vi "SubVI_Medicao.vi"(0 "Osciloscópio":refnum<visa-resource-name>="GPIB0::1::INSTR") -> (1 "Osciloscópio out":refnum<visa-resource-name>, 2 "Vmax":dbl, 3 "Vmin":dbl, 4 "Fase":dbl)   [LabVIEW 2021]
uses:
  384dc7f3-02c4-4d01-8472-58ff4c9df96a.vi
  292b6b08-2108-49e1-b5db-6c0617326701.vi
  c9bba13f-fd71-44bd-afed-ce225723edfd.vi
  4dd9f0b6-0c3f-4367-96f8-2e699b3ef568.vi
  dfb05754-934e-4608-8b12-f2cc72ba2c6f.vi
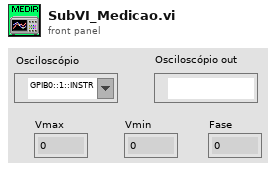
[diagram p1: front panel]
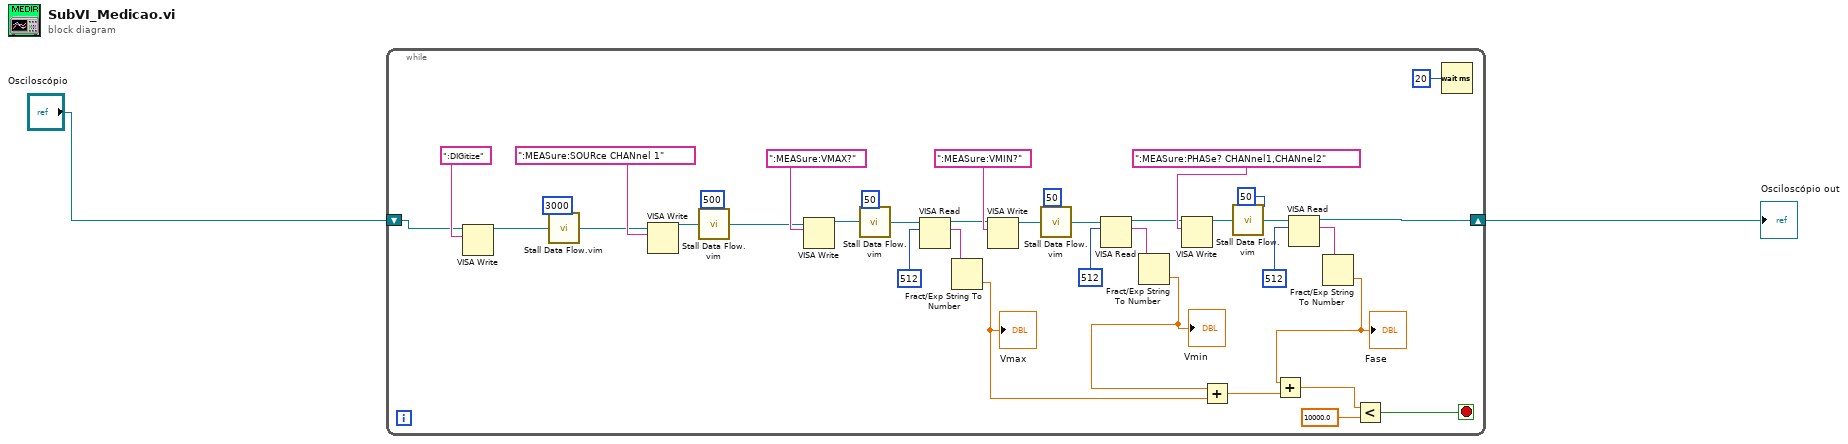
[diagram p0: block diagram]
diagram:
  n1 = while {
    shift-right: [w15] -> w2
    shift-left: "Osciloscópio" -> [w4]
    stop <- w24 stop-if-true
    n2 = VISA Write(VISA resource name=w4, write buffer=":DIGitize") -> (VISA resource name out=w5:refnum<visa-resource-name>)  [unwired: 1 in, 2 out]
    n3 = call "Stall Data Flow.vim"("value in"=w5, "milliseconds to wait"=u32 3000) -> ("value out"=w10:refnum<visa-resource-name>)  [unwired: 1 out]
    n4 = VISA Write(VISA resource name=w10, write buffer=":MEASure:SOURce CHANnel 1") -> (VISA resource name out=w7:refnum<visa-resource-name>)  [unwired: 1 in, 2 out]
    n5 = call "Stall Data Flow.vim"("value in"=w7, "milliseconds to wait"=u32 500) -> ("value out"=w3:refnum<visa-resource-name>)  [unwired: 1 out]
    n6 = VISA Write(VISA resource name=w3, write buffer=":MEASure:VMAX?") -> (VISA resource name out=w31:refnum<visa-resource-name>)  [unwired: 1 in, 2 out]
    n7 = call "Stall Data Flow.vim"("value in"=w31, "milliseconds to wait"=u32 50) -> ("value out"=w30:refnum<visa-resource-name>)  [unwired: 1 out]
    n8 = VISA Read(VISA resource name=w30, byte count=u32 512) -> (VISA resource name out=w36:refnum<visa-resource-name>, read buffer=w35:string)  [unwired: 1 in, 2 out]
    n9 = Fract/Exp String To Number(string=w35) -> (number=w26:dbl)  [unwired: 3 in, 1 out]
    "Vmax" <- w26
    n10 = VISA Write(VISA resource name=w36, write buffer=":MEASure:VMIN?") -> (VISA resource name out=w29:refnum<visa-resource-name>)  [unwired: 1 in, 2 out]
    n11 = call "Stall Data Flow.vim"("value in"=w29, "milliseconds to wait"=u32 50) -> ("value out"=w28:refnum<visa-resource-name>)  [unwired: 1 out]
    n12 = VISA Read(VISA resource name=w28, byte count=u32 512) -> (VISA resource name out=w16:refnum<visa-resource-name>, read buffer=w34:string)  [unwired: 1 in, 2 out]
    n13 = Fract/Exp String To Number(string=w34) -> (number=w27:dbl)  [unwired: 3 in, 1 out]
    "Vmin" <- w27
    n14 = VISA Write(VISA resource name=w16, write buffer=":MEASure:PHASe? CHANnel1,CHANnel2") -> (VISA resource name out=w22:refnum<visa-resource-name>)  [unwired: 1 in, 2 out]
    n15 = Add(x=w27, y=w26) -> (x+y=w14:dbl)
    n16 = call "Stall Data Flow.vim"("value in"=w22, "milliseconds to wait"=u32 50) -> ("value out"=w21:refnum<visa-resource-name>)  [unwired: 1 out]
    n17 = VISA Read(VISA resource name=w21, byte count=u32 512) -> (VISA resource name out=w15:refnum<visa-resource-name>, read buffer=w20:string)  [unwired: 1 in, 2 out]
    n18 = Fract/Exp String To Number(string=w20) -> (number=w13:dbl)  [unwired: 3 in, 1 out]
    "Fase" <- w13
    n19 = Add(x=w13, y=w14) -> (x+y=w12:dbl)
    n20 = Less?(x=w12, y=10000.0) -> (x < y?=w24:bool)
    n21 = Wait (ms)(milliseconds to wait=u32 20) -> ()  [unwired: 1 out]
  }
  "Osciloscópio out" <- w2
